vi "TW_Create.vi"(11 "Thingworx":string) -> (0 "Property out":string, 2 "Success?":bool)   [LabVIEW 2021]
panel:
  in  "Stop Button":bool
  in  "OK Button":bool
  in  "Type":u16(ring) items=["STRING", "NUMBER", "BOOLEAN", "IMAGE"]
  in  "Property":string
  out "Comm":T1
  # "Enter a name and type"
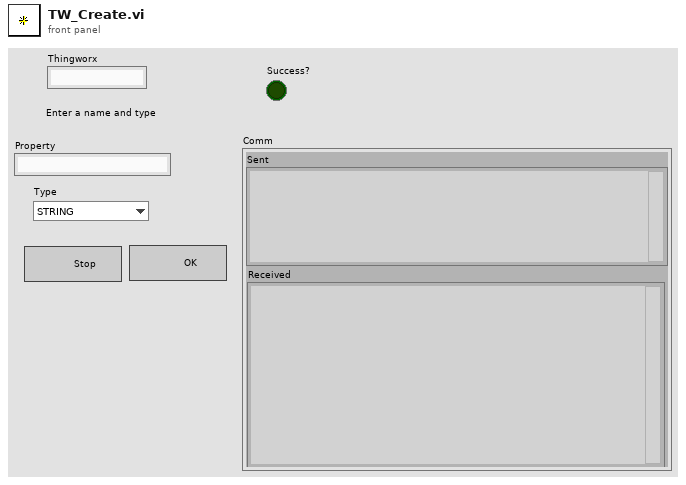
[diagram p1: front panel]
types:
  T1 = cluster{"url":string, "sent headers":string, "sent body":string, "headers":string, "body":string, "Sent":string, "Received":string}
  T2 = enum16{"GET", "PUT", "POST", "MultiPOST", "DELETE"}
  T3 = cluster{"name":string, "type":string, "logged":bool}
  T4 = cluster{"Name":string, "BaseURL":string, "AppKey":string, "Headers":string[], "Timeout":i32}
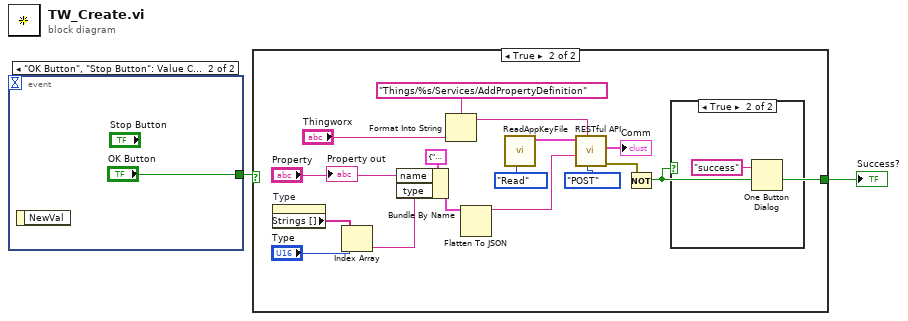
[diagram p0: block diagram]
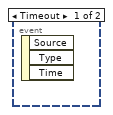
[diagram p4: hidden frame]
diagram:
  n1 = event shown="[1] \"OK Button\", \"Stop Button\": Value Change" {
    selector: _ -> [_ _]
    dyn-events: _ -> [_ _]
    timeout: _ -> [_ _]
    tunnel: [_ "OK Button"] -> w2
    event Timeout {
      n2 = event-data() -> ()  [unwired: 1 in, 3 out]
    }
    event "OK Button", "Stop Button": Value Change {
      n3 = event-data() -> ()  [unwired: 1 in, 1 out]
    }
  }
  n4 = case shown="True" w2 {
    tunnel: [_ w4] -> w1
    frame False {
    }
    frame True {
      n5 = property on="Type" class="Ring (strict)"() -> ("Strings []"=w8:string[])  [unwired: 2 in, 2 out]
      n6 = Index Array(array=w8, index="Type") -> (element=w6:string)
      n7 = Bundle By Name(cluster=T3 {"name"="", "type"="", "logged"=FALSE}, "name"="Property", "type"=w6) -> (w17:T3)
      n8 = Format Into String(format string="Things/%s/Services/AddPropertyDefinition", "Thingworx") -> (resulting string=w15:string)  [unwired: 2 in, 1 out]
      n9 = Flatten To JSON(anything=w17) -> (JSON string=w12:string)  [unwired: 2 in, 1 out]
      n10 = call "ReadAppKeyFile.vi"("Task"=enum16{"Read", "Write"}."Read") -> ("Device Out"=w13:T4)  [unwired: 8 in, 2 out]
      n11 = call "RESTful API.vi"("Method"=T2."POST", "url"=w15, "JSON"=w12, "Device In"=w13) -> ("error out"=w10:errorcluster, "Comm"=→"Comm":T1)  [unwired: 5 in, 1 out]
      n12 = Not(x=w10) -> (.not. x?=w4:bool)
      n13 = case shown="True" w4 {
        frame False {
        }
        frame True {
          n14 = One Button Dialog(message="success") -> ()  [unwired: 1 in, 1 out]
        }
      }
      "Property out" <- "Property"
    }
  }
  "Success?" <- w1
